vi "Run.vi"() -> ()   [LabVIEW 2018]
panel:
  out "VI Name 2":string
  out "Numeric":i32
  out "Application:All VIs In Memory":string[](array[string])
  out "Time":u32
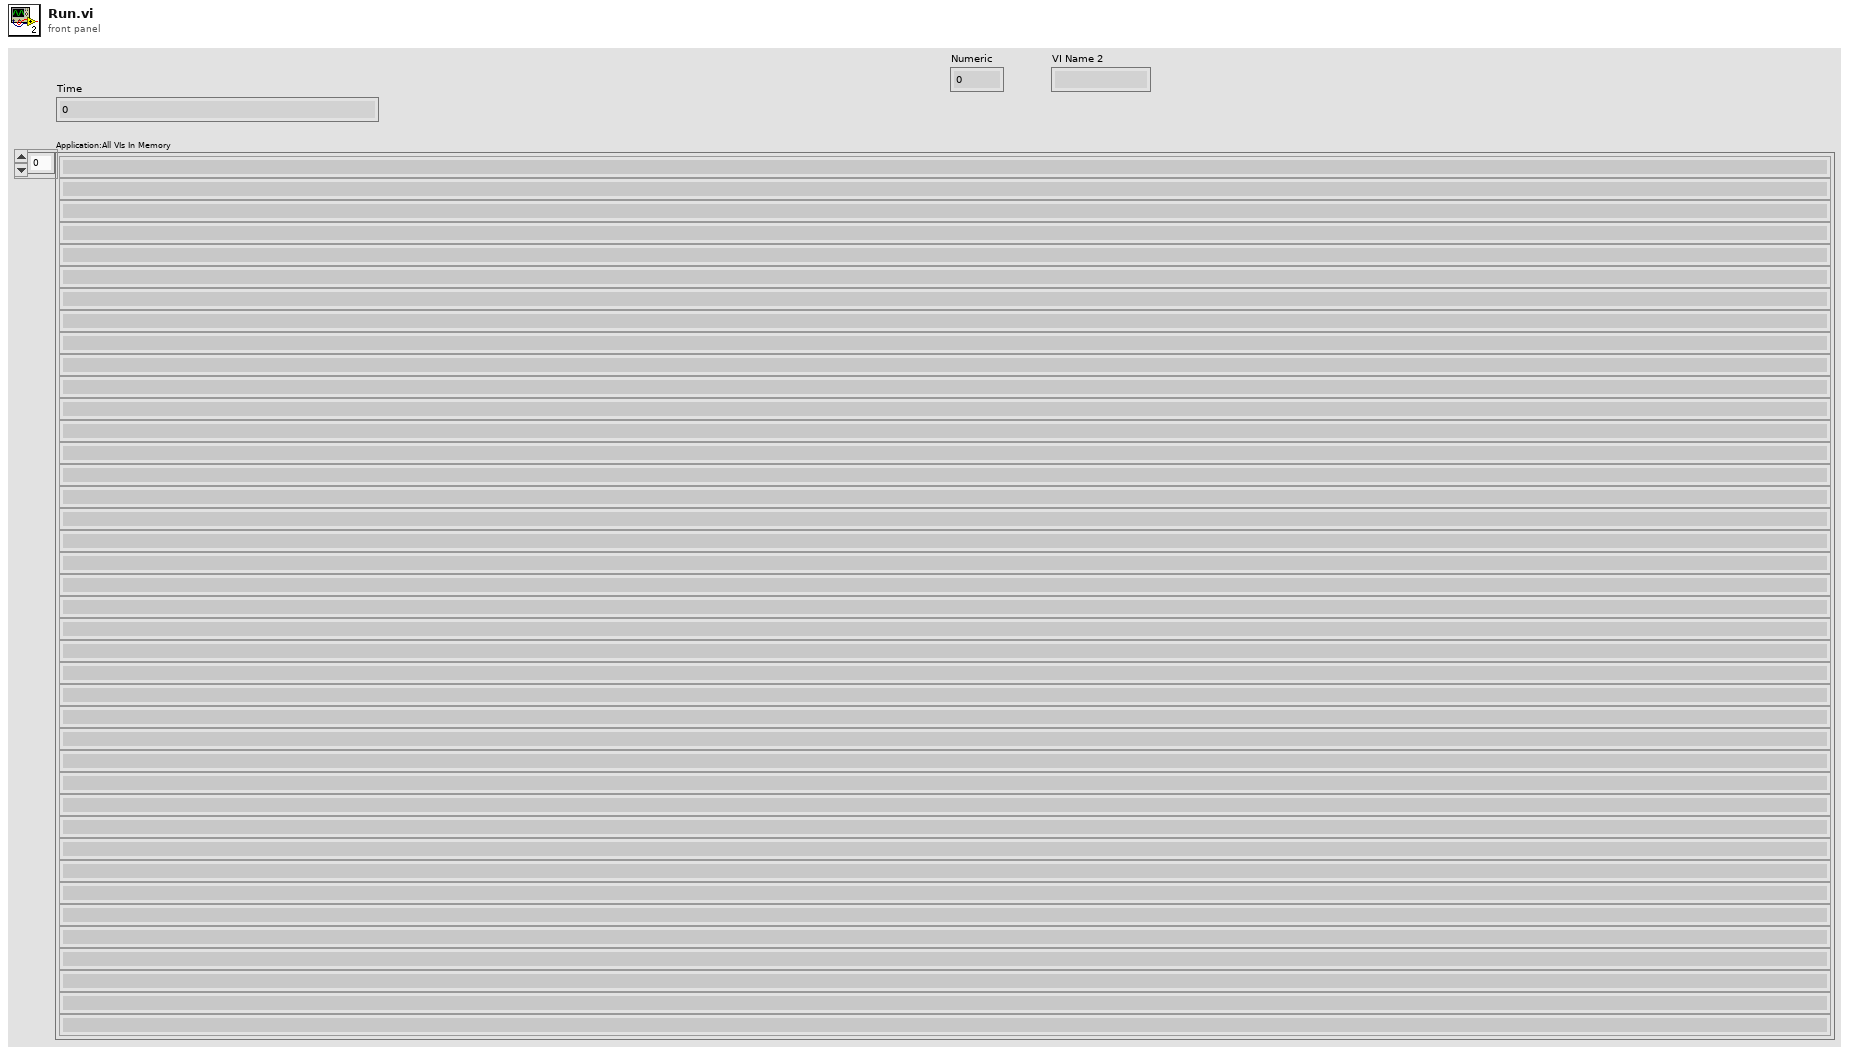
[diagram p1: front panel]
types:
  T1 = enum32{"Invalid", "Standard", "Closed", "Hidden", "Minimized", "Maximized"}
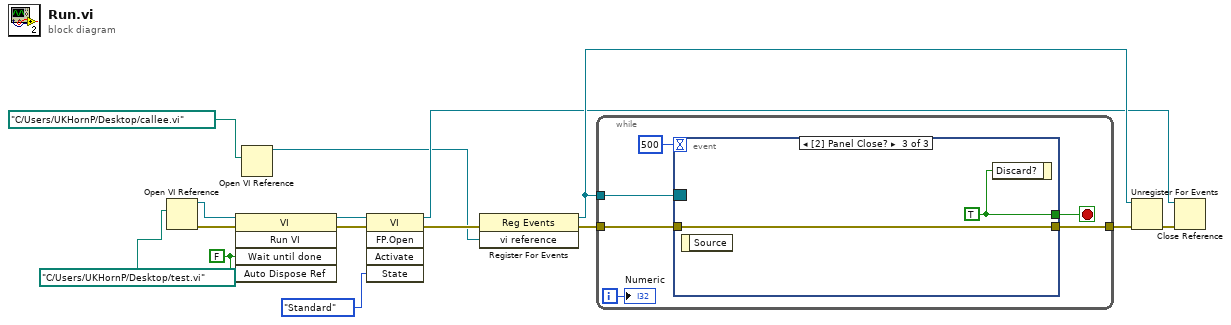
[diagram p0: block diagram]
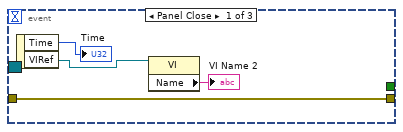
[diagram p2: hidden frame]
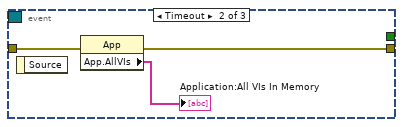
[diagram p3: hidden frame]
diagram:
  w12 = FALSE ("Wait Until Done")
  n1 = Open VI Reference(vi path=path "C:/Users/UKHornP/Desktop/test.vi" ("VI Path")) -> (vi reference=w14:refnum<vi>, error out=w13:errorcluster)  [unwired: 5 in]
  n2 = invoke class="VI" method="Run VI"(reference=w14, error in=w13, "Wait until done"=w12, "Auto Dispose Ref"=w12) -> (reference out=w6:refnum<vi>, error out=w11:errorcluster)  [unwired: 1 in, 3 out]
  n3 = Open VI Reference(vi path=path "C:/Users/UKHornP/Desktop/callee.vi" ("VI Path")) -> (vi reference=w1:refnum<vi>)  [unwired: 5 in, 1 out]
  n4 = invoke class="VI" method="FP.Open"(reference=w6, error in=w11, "State"=T1."Standard") -> (reference out=w3:refnum<vi>, error out=w7:errorcluster)  [unwired: 2 in, 3 out]
  n5 = register-events(error in=w7, w1) -> (reference out=w9:refnum<event-registration>, error out=w4:errorcluster)  [unwired: 1 in]
  n6 = while {
    tunnel: w4 -> [w21]
    tunnel: w9 -> [w20]
    tunnel: [w18] -> w10
    i -> [w16]
    stop <- w19 stop-if-true
    n7 = event shown="[2] Panel Close?" {
      selector: w20 -> [_ _ _]
      dyn-events: _ -> [_ _ _]
      timeout: 500 -> [_ _ _]
      tunnel: w21 -> [w24 w28 w29]
      tunnel: [_ _ w30] -> w19
      tunnel: [w24 w26 w29] -> w18
      event Panel Close {
        n8 = event-data() -> ("Time"=→"Time":u32, "VIRef"=w23:refnum<vi>)  [unwired: 1 in]
        n9 = property class="VI"(reference=w23) -> ("Name"=→"VI Name 2":string)  [unwired: 1 in, 2 out]
      }
      event Timeout {
        n10 = event-data() -> ()  [unwired: 1 in, 1 out]
        n11 = property class="App"(error in=w28) -> (error out=w26:errorcluster, "App.AllVIs"=→"Application:All VIs In Memory":string[])  [unwired: 1 in, 1 out]
      }
      event Panel Close? {
        w30 = TRUE ("Discard?")
        n12 = event-data() -> ()  [unwired: 1 in, 1 out]
        n13 = event-data("Discard?"=w30) -> ()  [unwired: 1 in, 1 out]
      }
    }
    "Numeric" <- w16
  }
  n14 = Unregister For Events(event registration refnum=w9, error in=w10) -> (error out=w8:errorcluster)
  n15 = Close Reference(reference=w3, error in (no error)=w8) -> ()  [unwired: 1 out]
